vi "LPCA Interface Front Panel Update.vi"(6 "Resistance":refnum<vi>, 7 "index":i32, 8 "error in (no error)":errorcluster, 9 "Cluster":T1={"Queue Array"=[], "Queue Element"={"state"="", "data"=variant}, "System Event"=refnum, "System Event RefNum"=refnum, "Queue List"=[], "LPCA COM"="", "Rotating"=FALSE, "PrecorAI"="", "T_0 Index"=0, "Bar Graph X"=[], "Channels"=[], "Active Indicies"=[], "Active Channels"=[], "Sample Frequency"=0.0, "Resistance Sweep"=[], "RPM Sweep"=[], "Load Sweep"=[], "Step Height Sweep"=[], "Range Sweep"=[], "A Counter"=0, "B Counter"=0, "C Counter"=0, "#A"=0, "#B"=0, "#C"=0, "Current RPM"=0.0, "Current Resistance"=0, "Current Range"=0, "Current Step Height"=0, "Load Bank"=enum."OFF", "Cfg Cntrls"=[], "T_Monitor Indices"=[], "Thermal Limit"=0, "Thermal Resume"=0, "Timer Reset"=FALSE, "Stop Time"=0.0, "Autotest"=FALSE, "Pulsed RPM Capture"=FALSE, "Get Sample"=FALSE, "Last State"="", "Reset Timeout"=FALSE, "Ctrl Refs"={"Test Details"=refnum, "Save Config"=refnum, "Load Config"=refnum, "Path"=refnum, "Snapshot"=refnum, "SS#"=refnum, "Resistance"=refnum, "RPM Target"=refnum, "Spin"=refnum, "Load Bank"=refnum, "Start Test"=refnum, "Pause Test"=refnum, "Load Sweep"=refnum, "RPM Sweep"=refnum, "Resistance Sweep"=refnum, "Filters"=refnum, "Sample Frequency"=refnum, "Data Setup"=refnum, "Pause"=refnum, "Stop Time"=refnum, "S Period"=refnum, "Range"=refnum, "Step Height"=refnum, "Step Height Sweep"=refnum, "Range Sweep"=refnum, "Available Tests"=refnum, "RPM Graph"=refnum, "RPM Knob"=refnum, "FanMode"=refnum, "Fan Mode LED Array"=refnum, "Thermal Equilibrium"=refnum, "Data Display"=refnum, "LPCA Error"=refnum, "LPCA Ramp"=refnum, "LPCA Range"=refnum, "LPCA Resistance"=refnum}, "Pulse Waveform"={"t0"=timestamp(0 s since 1904-01-01), "dt"=1.0, "Y"=[]}, "Snapshot"={"Test Details"="test", "Version"="test", "Date"=timestamp(3493915594.3018084 s since 1904-01-01), "Selected Test"="man", "Snapshot Number"=0, "Time"=timestamp(3493915602.7292905 s since 1904-01-01), "Resistance Setpoint"="1", "RPM Setpoint"="20", "Range Setpoint"="", "Step Height Setpoint"="", "Load Bank Setpoint"="15", "Measurement Headers"="a,b,c,1,2,3", "Measurements"="1,2,3,4,5,6,7,8", "A"=0, "B"=0, "C"=0, "Raw Data"=[], "Available Tests"=enum."Manual", "Resistance List"="", "RPM List"="", "Load Bank List"="", "Range List"="", "Step Height List"="", "FanMode Setpoint"=enum."Auto"}, "Sample Period"=0.0, "OverTemp"=FALSE, "Available Tests"=enum."Manual", "FanMode"=enum."Auto", "Fan Mode LED Array"=[FALSE, TRUE, FALSE], "Thermal\nEquilibrium "=FALSE, "Equilibrium Stop"=FALSE, "AvgDegChg"=[]} {"Snapshot"."Time" format="%<%H:%M:%S>T"; "Snapshot"."Date" format="%<%m/%d/%Y>T"}, 10 "String":refnum<vi>) -> ()   [LabVIEW 2017]
uses:
  Controls/LPCA Commands.ctl
  <vilib>/regexp/Match Regular Expression.xnode
  <vilib>/Instr/_visa.llb/VISA Configure Serial Port (Instr).vi
  Code Library/Queue Element.ctl
  Code Library/Queue References Array.ctl
  Controls/Test TypeDef.ctl
  Controls/Available Tests.ctl
  Controls/Snapshot Typedef.ctl
  Controls/Load Bank.ctl
  Controls/FanMode.ctl
panel:
  out "return count":u32
  out "Stop?":bool=TRUE
  out "VISA resource name out":refnum<visa-resource-name>
  out "before match":string
  out "number of replacements":i32
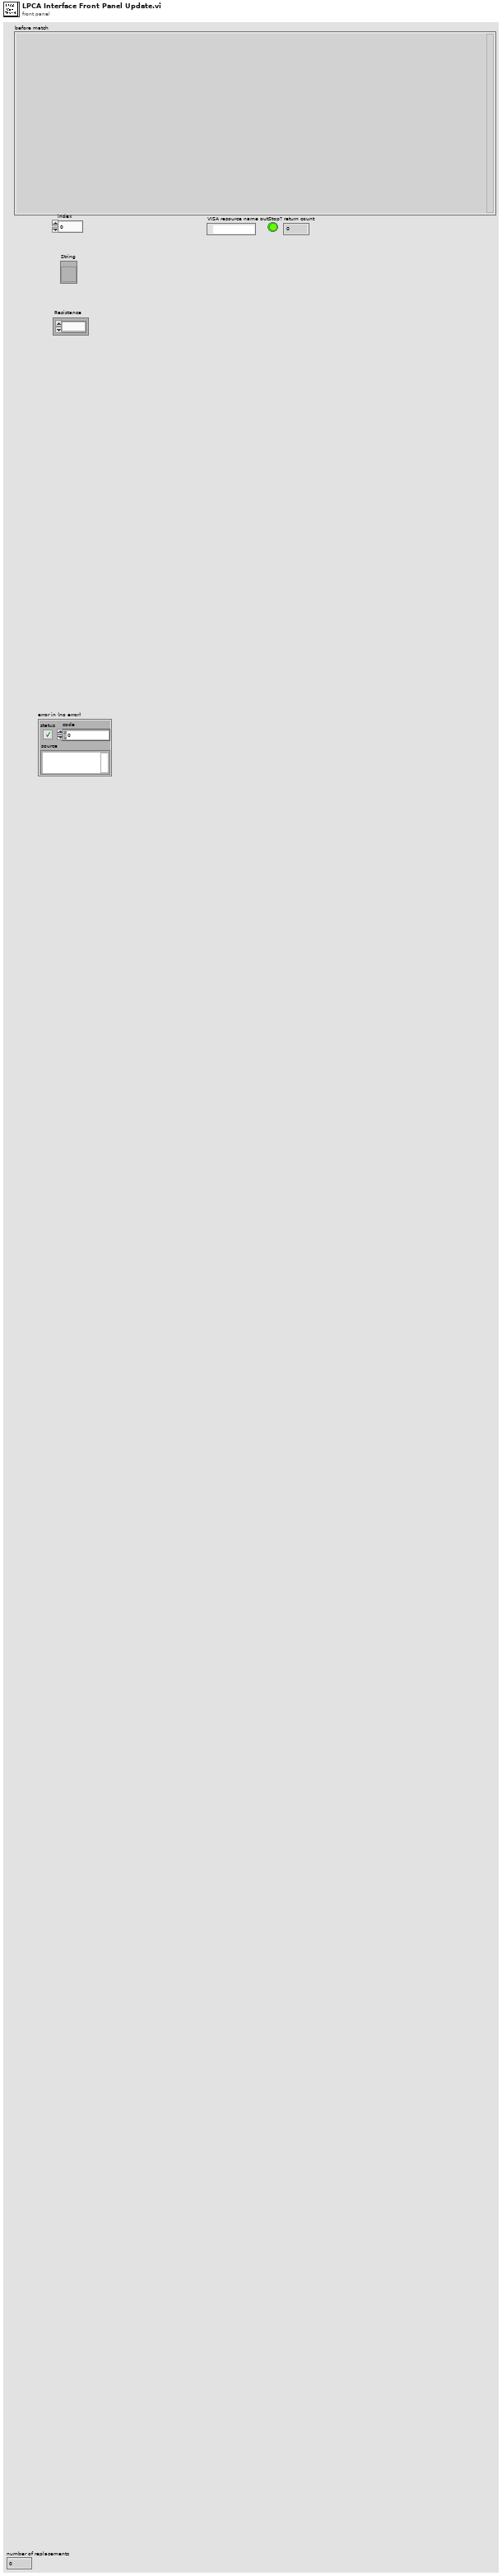
[diagram p1: front panel]
types:
  T1 = typedef "Test TypeDef.ctl" = cluster{"Queue Array":T2, "Queue Element":T3, "System Event":refnum<user-event>, "System Event RefNum":refnum<event-registration>, "Queue List":string[], "LPCA COM":refnum<visa-resource-name>, "Rotating":bool, "PrecorAI":refnum<k21>, "T_0 Index":i32, "Bar Graph X":i32[], "Channels":string[], "Active Indicies":i32[], "Active Channels":string[][], "Sample Frequency":dbl, "Resistance Sweep":string[], "RPM Sweep":string[], "Load Sweep":string[], "Step Height Sweep":string[], "Range Sweep":string[], "A Counter":i32, "B Counter":i32, "C Counter":i32, "#A":i32, "#B":i32, "#C":i32, "Current RPM":dbl, "Current Resistance":u32, "Current Range":u32, "Current Step Height":u32, "Load Bank":T4, "Cfg Cntrls":refnum<vi>[], "T_Monitor Indices":i32[], "Thermal Limit":i32, "Thermal Resume":i32, "Timer Reset":bool, "Stop Time":dbl, "Autotest":bool, "Pulsed RPM Capture":bool, "Get Sample":bool, "Last State":string, "Reset Timeout":bool, "Ctrl Refs":cluster{"Test Details":refnum<vi>, "Save Config":refnum<vi>, "Load Config":refnum<vi>, "Path":refnum<vi>, "Snapshot":refnum<vi>, "SS#":refnum<vi>, "Resistance":refnum<vi>, "RPM Target":refnum<vi>, "Spin":refnum<vi>, "Load Bank":refnum<vi>, "Start Test":refnum<vi>, "Pause Test":refnum<vi>, "Load Sweep":refnum<vi>, "RPM Sweep":refnum<vi>, "Resistance Sweep":refnum<vi>, "Filters":refnum<vi>, "Sample Frequency":refnum<vi>, "Data Setup":refnum<vi>, "Pause":refnum<vi>, "Stop Time":refnum<vi>, "S Period":refnum<vi>, "Range":refnum<vi>, "Step Height":refnum<vi>, "Step Height Sweep":refnum<vi>, "Range Sweep":refnum<vi>, "Available Tests":refnum<vi>, "RPM Graph":refnum<vi>, "RPM Knob":refnum<vi>, "FanMode":refnum<vi>, "Fan Mode LED Array":refnum<vi>, "Thermal Equilibrium":refnum<vi>, "Data Display":refnum<vi>, "LPCA Error":refnum<vi>, "LPCA Ramp":refnum<vi>, "LPCA Range":refnum<vi>, "LPCA Resistance":refnum<vi>}, "Pulse Waveform":waveform(dbl), "Snapshot":T5, "Sample Period":dbl, "OverTemp":bool, "Available Tests":T6, "FanMode":T7, "Fan Mode LED Array":bool[], "Thermal\nEquilibrium ":bool, "Equilibrium Stop":bool, "AvgDegChg":dbl[]}
  T2 = typedef "Queue References Array.ctl" = refnum<queue>[]
  T3 = typedef "Queue Element.ctl" = cluster{"state":string, "data":variant}
  T4 = typedef "Load Bank.ctl" = enum16{"OFF", "50", "25", "16.7", "12.5", "10.0", "8.3", "7.1", "6.3", "5.6", "5.0", "4.5", "4.2", "3.8", "3.6", "3.3", "3.1"}
  T5 = typedef "Snapshot Typedef.ctl" = cluster{"Test Details":string, "Version":string, "Date":timestamp, "Selected Test":string, "Snapshot Number":u16, "Time":timestamp, "Resistance Setpoint":string, "RPM Setpoint":string, "Range Setpoint":string, "Step Height Setpoint":string, "Load Bank Setpoint":string, "Measurement Headers":string, "Measurements":string, "A":i32, "B":i32, "C":i32, "Raw Data":string[][], "Available Tests":T6, "Resistance List":string, "RPM List":string, "Load Bank List":string, "Range List":string, "Step Height List":string, "FanMode Setpoint":T7}
  T6 = typedef "Available Tests.ctl" = enum16{"Manual", "EFX Brake Torque", "Generator Torque", "EFX Brake Thermal", "Generator Thermal", "Pulsed RPM", "AMT Brake Torque", "Bike Brake Torque", "AMT Brake Thermal", "Bike Brake Thermal"}
  T7 = typedef "FanMode.ctl" = enum16{"On", "Off", "Auto"}
  T8 = typedef "LPCA Commands.ctl" = enum16{"RSET", "stop", "rpmh", "rpml", "prpm", "rpm", "res", "rng", "tmp1", "tmp2", "err", "ramp"}
  T9 = cluster{"Test Details":refnum<vi>, "Save Config":refnum<vi>, "Load Config":refnum<vi>, "Path":refnum<vi>, "Snapshot":refnum<vi>, "SS#":refnum<vi>, "Resistance":refnum<vi>, "RPM Target":refnum<vi>, "Spin":refnum<vi>, "Load Bank":refnum<vi>, "Start Test":refnum<vi>, "Pause Test":refnum<vi>, "Load Sweep":refnum<vi>, "RPM Sweep":refnum<vi>, "Resistance Sweep":refnum<vi>, "Filters":refnum<vi>, "Sample Frequency":refnum<vi>, "Data Setup":refnum<vi>, "Pause":refnum<vi>, "Stop Time":refnum<vi>, "S Period":refnum<vi>, "Range":refnum<vi>, "Step Height":refnum<vi>, "Step Height Sweep":refnum<vi>, "Range Sweep":refnum<vi>, "Available Tests":refnum<vi>, "RPM Graph":refnum<vi>, "RPM Knob":refnum<vi>, "FanMode":refnum<vi>, "Fan Mode LED Array":refnum<vi>, "Thermal Equilibrium":refnum<vi>, "Data Display":refnum<vi>, "LPCA Error":refnum<vi>, "LPCA Ramp":refnum<vi>, "LPCA Range":refnum<vi>, "LPCA Resistance":refnum<vi>}
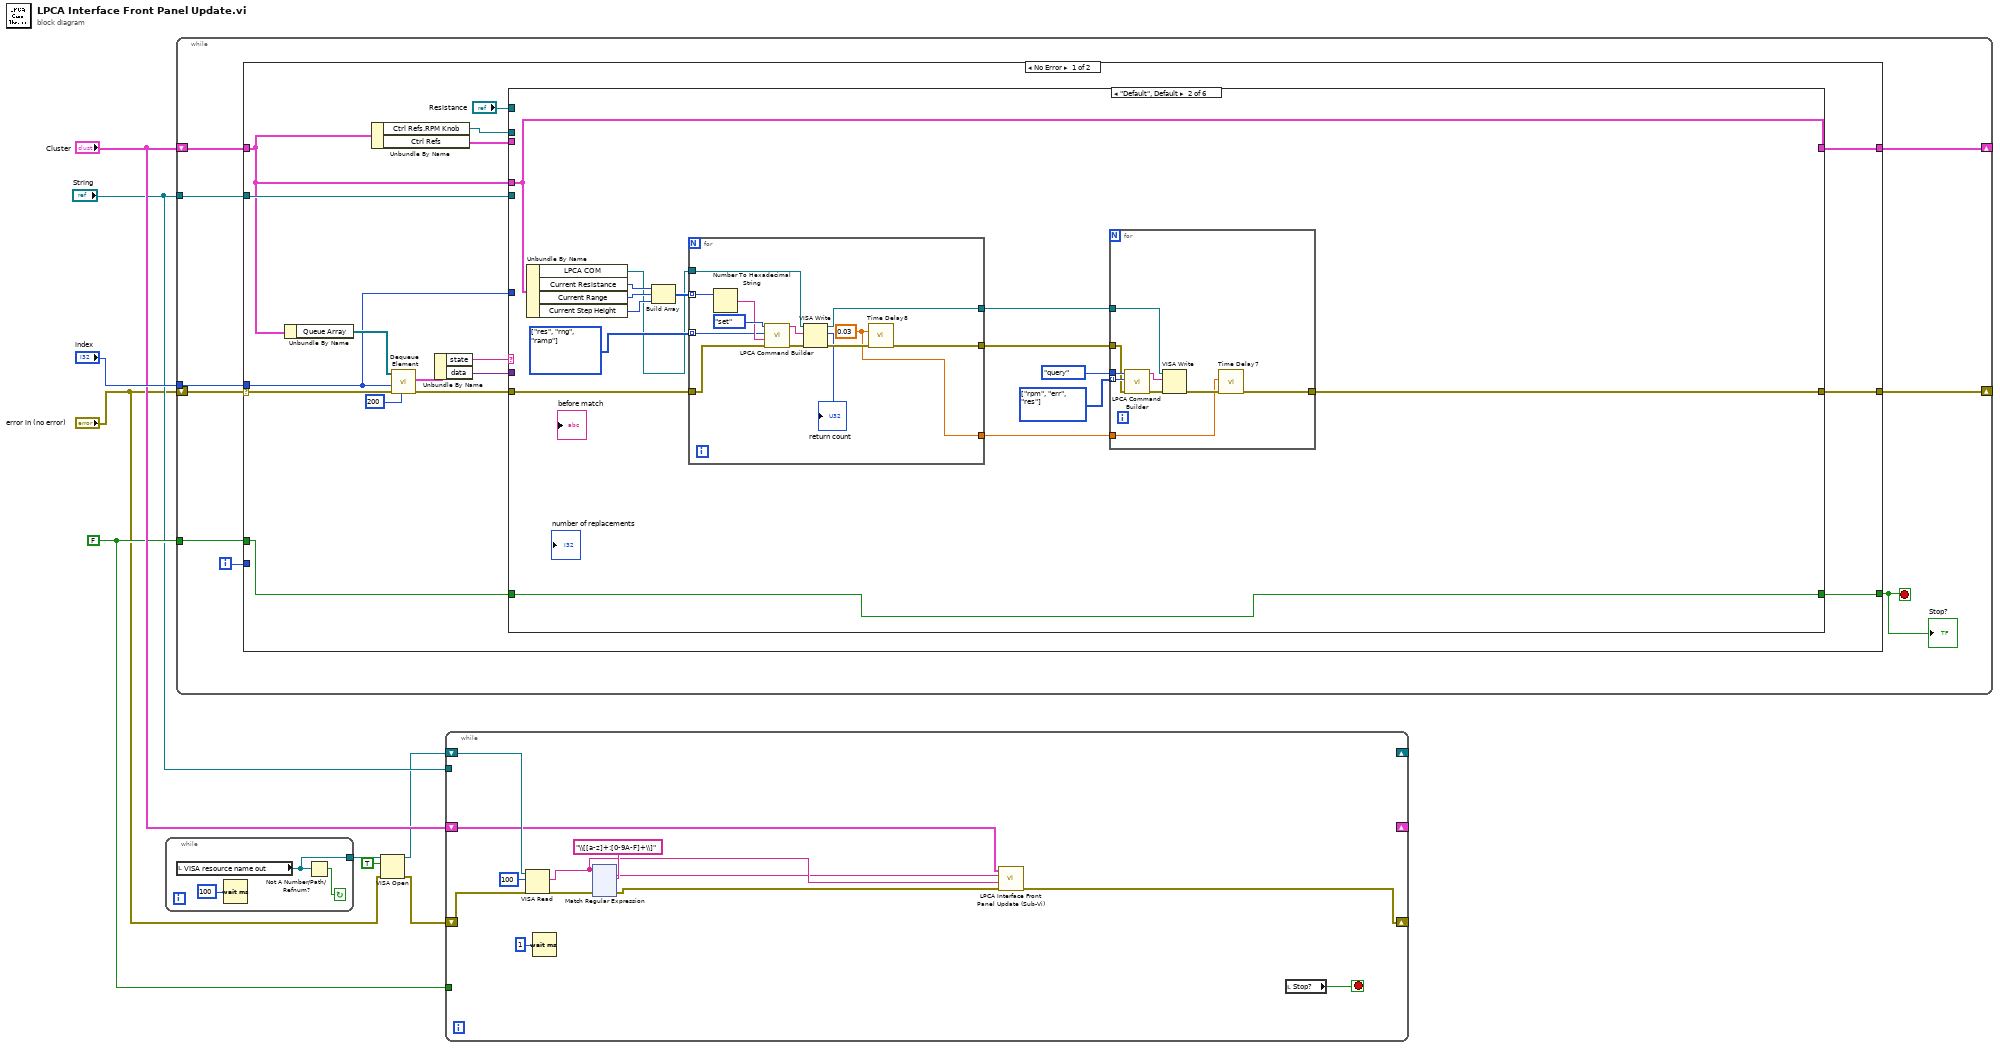
[diagram p0: block diagram]
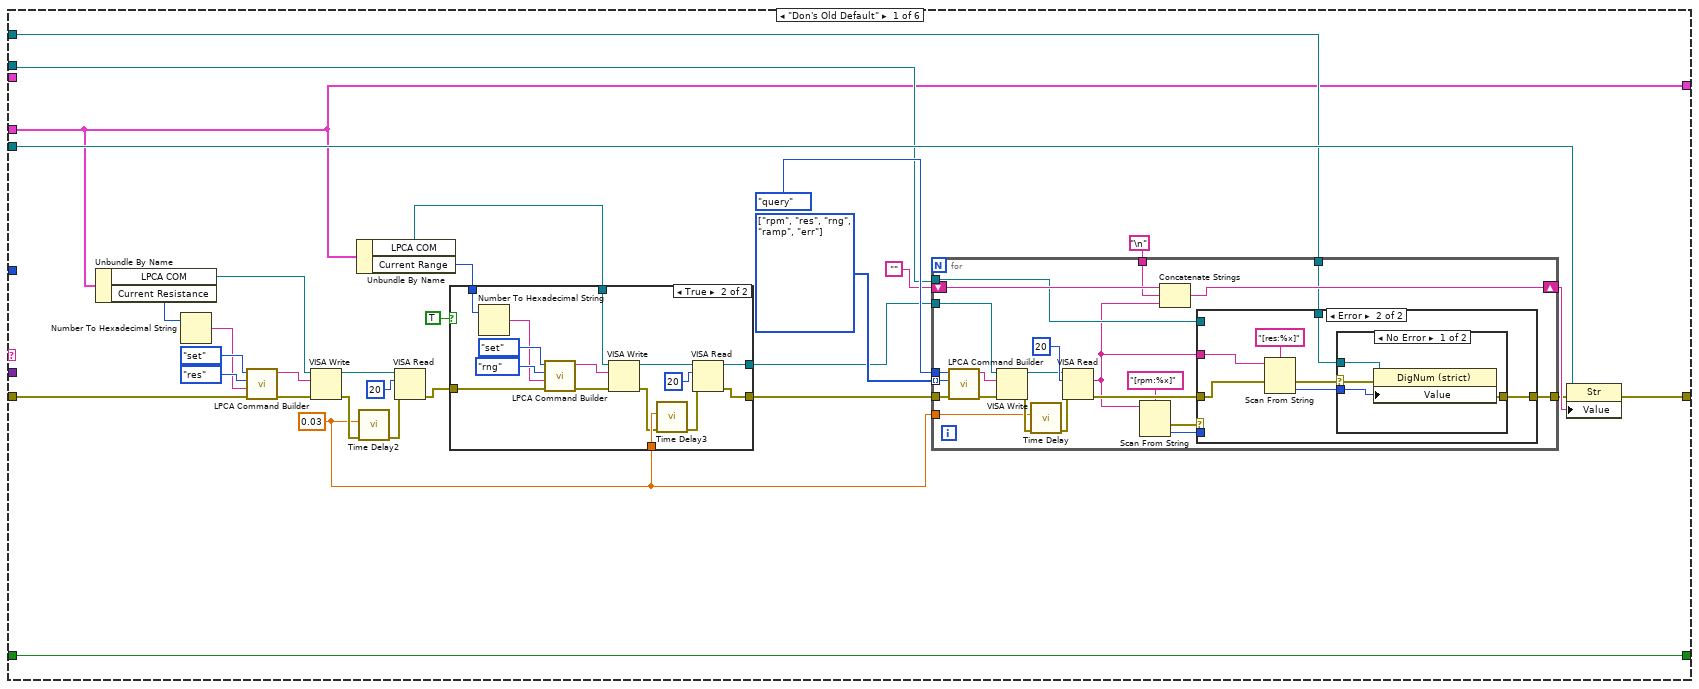
[diagram p2: hidden frame]
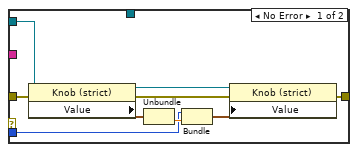
[diagram p4: hidden frame]
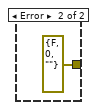
[diagram p5: hidden frame]
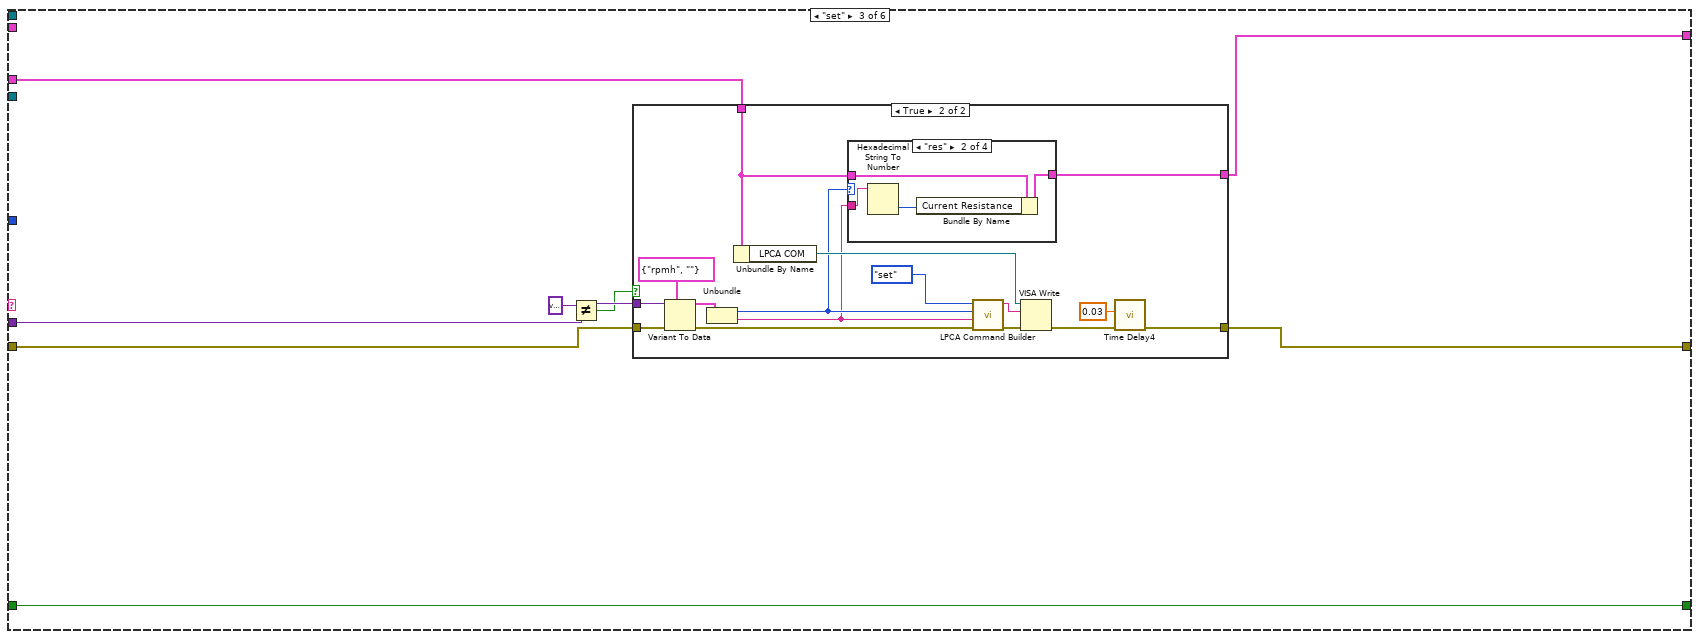
[diagram p6: hidden frame]
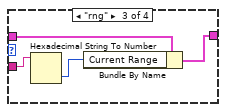
[diagram p9: hidden frame]
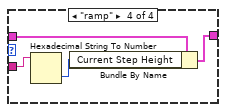
[diagram p10: hidden frame]
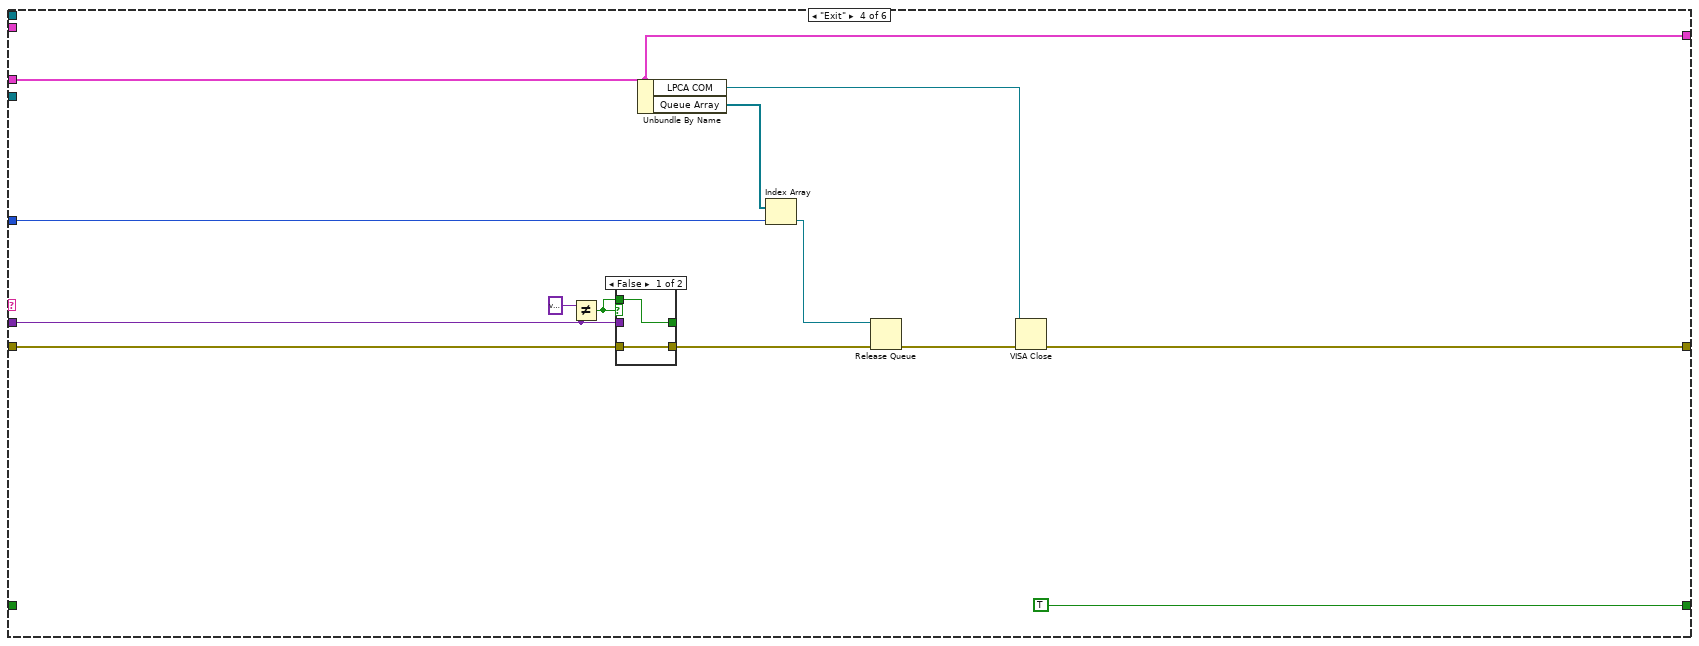
[diagram p11: hidden frame]
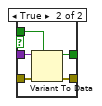
[diagram p12: hidden frame]
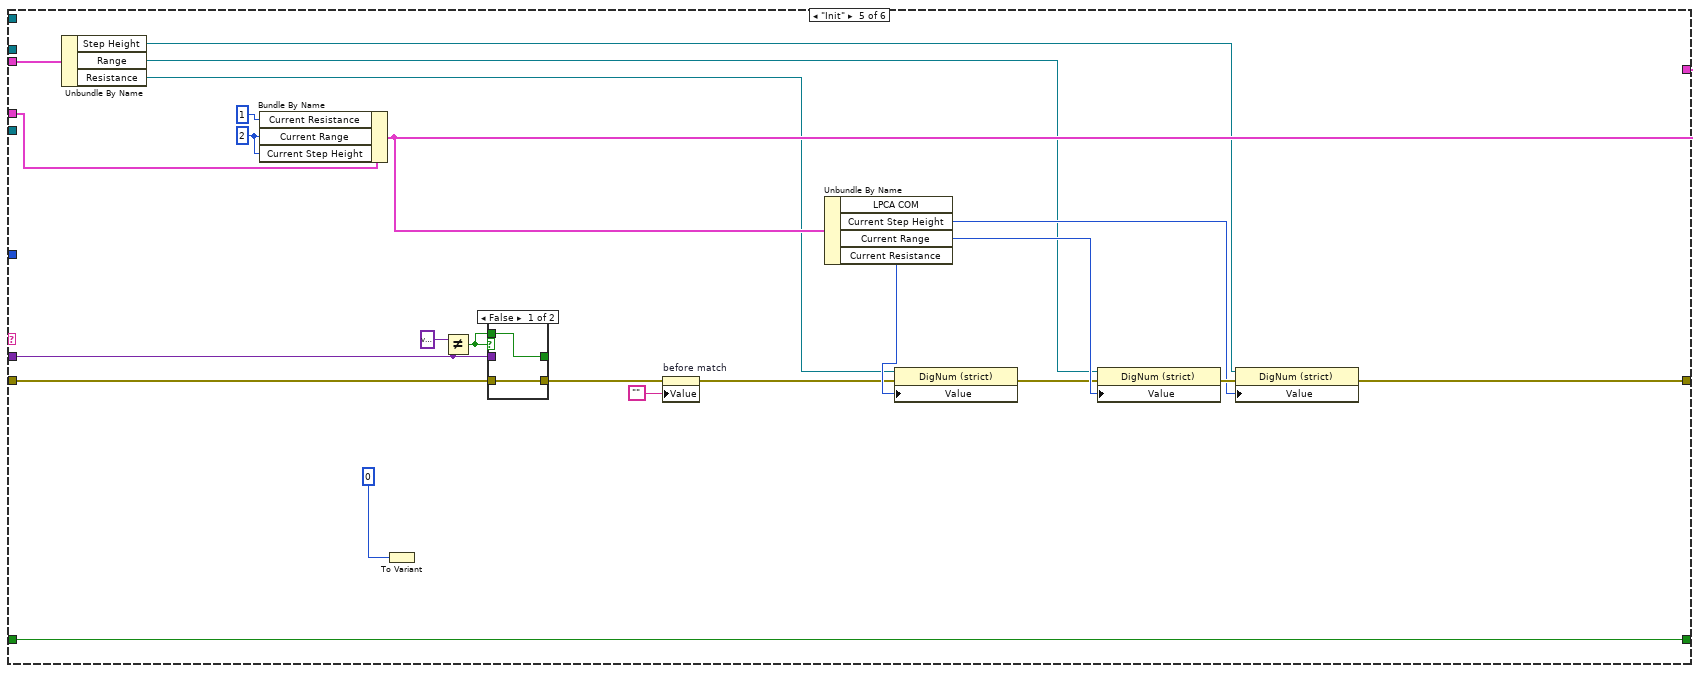
[diagram p13: hidden frame]
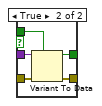
[diagram p14: hidden frame]
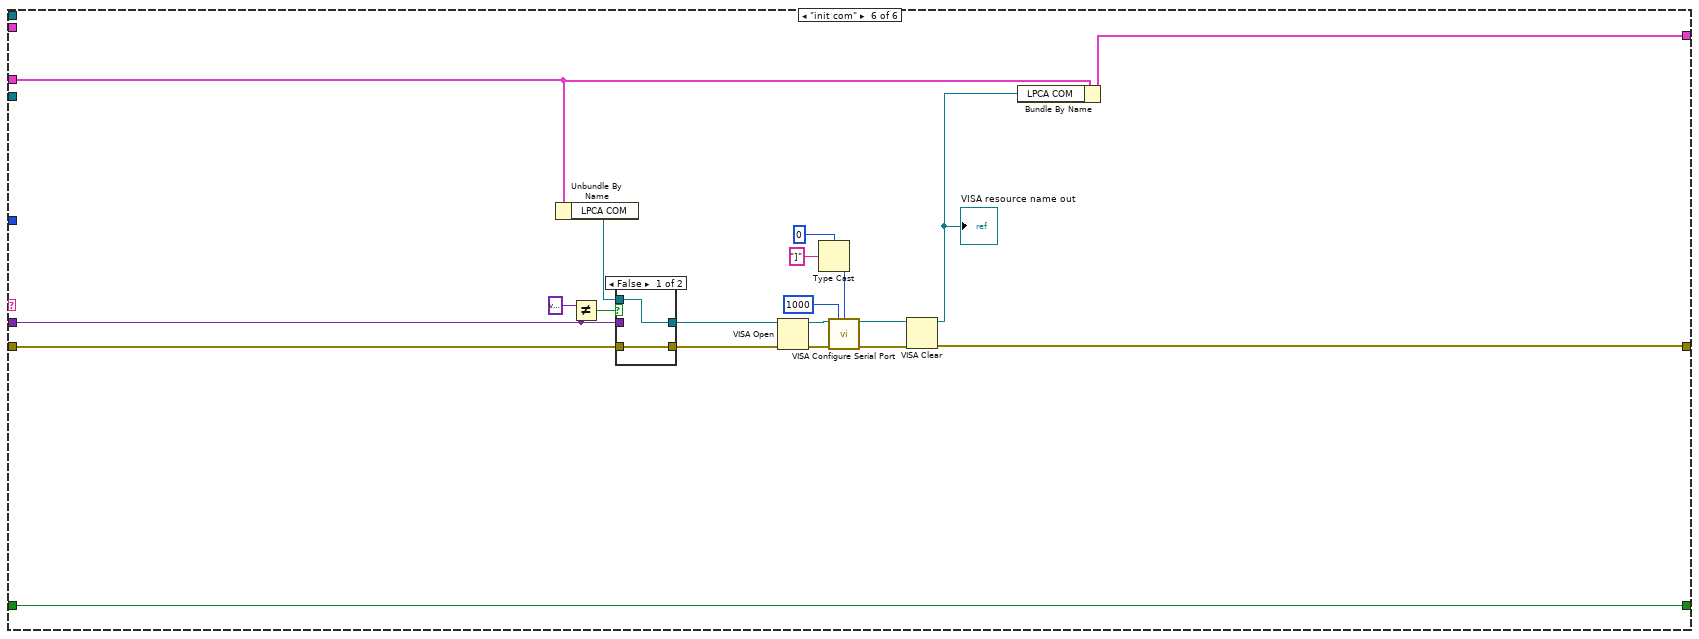
[diagram p15: hidden frame]
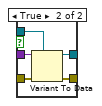
[diagram p16: hidden frame]
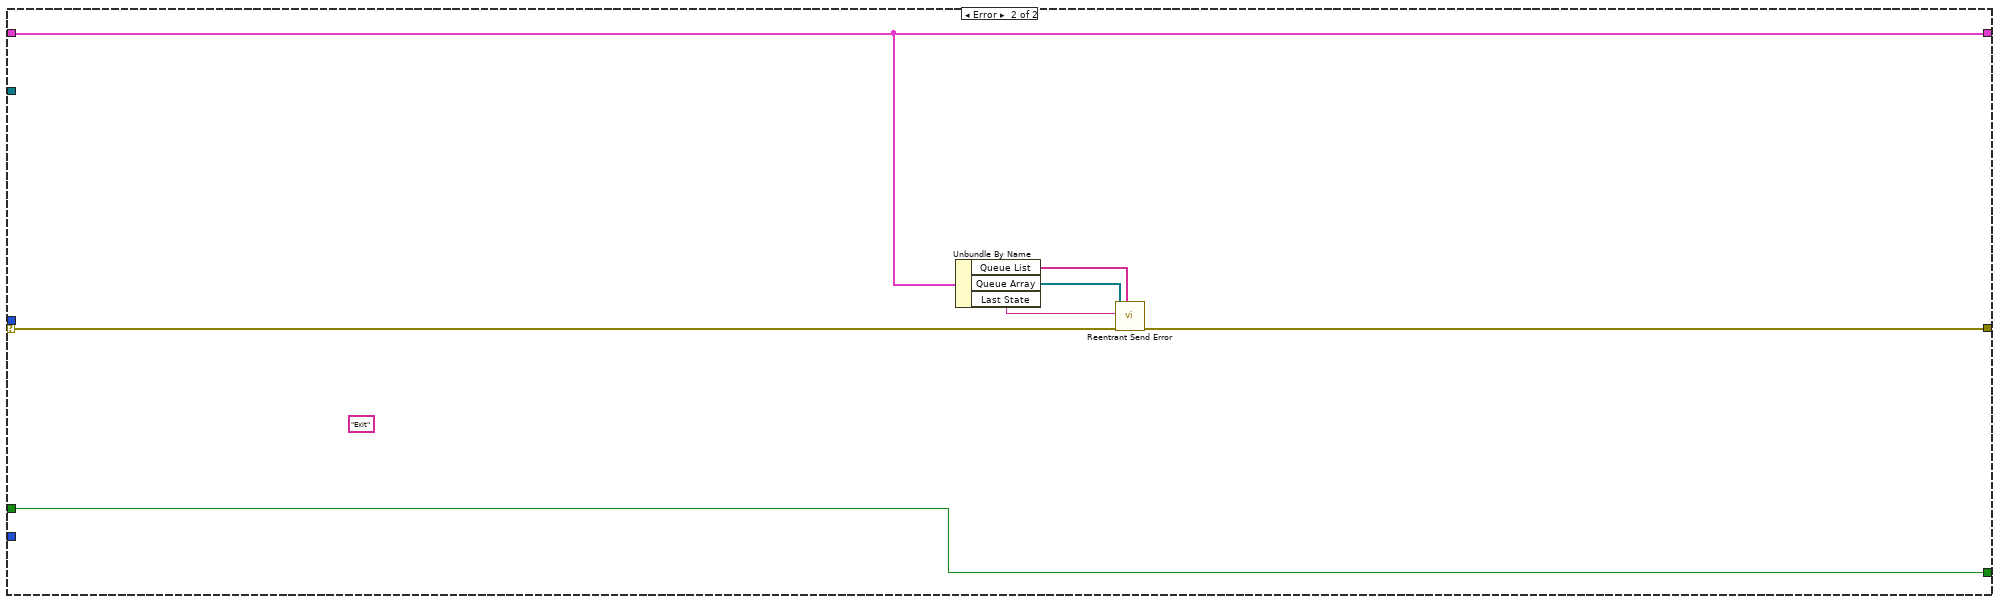
[diagram p17: hidden frame]
diagram:
  w7 = FALSE ("Boolean")
  n1 = while {
    tunnel: [w10] -> w5
    stop <- w11 continue-if-true
    n2 = local read "VISA resource name out"() -> (w10:refnum<visa-resource-name>)
    n3 = Wait (ms)(milliseconds to wait=u32 100) -> ()  [unwired: 1 out]
    n4 = Not A Number/Path/Refnum?(number/path/refnum=w10) -> (NaN/Path/Refnum?=w11:bool)
  }
  n5 = while {
    shift-right: [w17] -> _
    shift-left: "Cluster" -> [w21]
    tunnel: w7 -> [w18]
    shift-right: [w19] -> _
    shift-left: "error in (no error)" -> [w20]
    tunnel: "index" -> [w16]
    tunnel: "String" -> [w15]
    i -> [w14]
    stop <- w13 stop-if-true
    n6 = case shown="No Error" w20 {
      selector: w20 -> [w36 w285]
      tunnel: w21 -> [w23 w283]
      tunnel: [w34 w284] -> w19
      tunnel: w18 -> [w33 w289]
      tunnel: [w32 w289] -> w13
      tunnel: [w30 w283] -> w17
      tunnel: w16 -> [w26 _]
      tunnel: w15 -> [w29 _]
      tunnel: w14 -> [_ _]
      frame No Error {
        n7 = Unbundle By Name(w23) -> ("Queue Array"=w38:T2)
        n8 = Unbundle By Name(w23) -> ("Ctrl Refs.RPM Knob"=w25:refnum<vi>, "Ctrl Refs"=w24:T9)
        n9 = call "Dequeue Element.vi"("timeout in ms (-1)"=200, "error in (no error)"=w36, "index"=w26, "Queue Array"=w38) -> ("error out"=w35:errorcluster, "Queue Element"=w28:T3)  [unwired: 5 in, 1 out]
        n10 = Unbundle By Name(w28) -> ("state"=w22:string, "data"=w31:variant)
        n11 = case shown="\"Default\", Default" w22 {
          tunnel: w35 -> [w49 w133 w173 w218 w247 w274]
          tunnel: [w68 w130 w170 w211 w226 w256] -> w34
          tunnel: w33 -> [w69 w144 w174 _ w248 w275]
          tunnel: [w69 w144 w174 TRUE ("Boolean") w248 w275] -> w32
          tunnel: w31 -> [_ _ w171 w216 w245 w272]
          tunnel: [w43 w132 w167 w214 w236 w270] -> w30
          tunnel: w23 -> [w43 w132 w168 w214 w239 w262]
          tunnel: w29 -> [w66 _ _ _ _ _]
          tunnel: w25 -> [w48 _ _ _ _ _]
          tunnel: "Resistance" -> [w47 _ _ _ _ _]
          tunnel: w26 -> [_ _ _ w208 _ _]
          tunnel: w24 -> [_ _ _ _ w235 _]
          frame "Don's Old Default" {
            w53 = T8[] [enum."rpm", enum."res", enum."rng", enum."ramp", enum."err"] items=["RSET", "stop", "rpmh", "rpml", "prpm", "rpm", "res", "rng", "tmp1", "tmp2", "err", "ramp"]
            w46 = 0.03 ("Delay Time (s)")
            n12 = Unbundle By Name(w43) -> ("LPCA COM"=w67:refnum<visa-resource-name>, "Current Resistance"=w65:u32)
            n13 = Number To Hexadecimal String(2:w65) -> (0:w55:string)  [unwired: 1 in]
            n14 = call "LPCA Command Builder.vi"("error in (no error)"=w49, "Data"=w55, "LPCA Command"=LPCA_Commands."res", "Mode"=enum16{"set", "query"}."set") -> ("error out"=w56:errorcluster, "String"=w57:string)  [unwired: 6 in]
            n15 = VISA Write(VISA resource name=w67, write buffer=w57, error in (no error)=w56) -> (VISA resource name out=w51:refnum<visa-resource-name>, error out=w54:errorcluster)  [unwired: 1 out]
            n16 = Unbundle By Name(w43) -> ("LPCA COM"=w41:refnum<visa-resource-name>, "Current Range"=w44:u32)
            n17 = call "Time Delay2"("error in (no error)"=w54, "Delay Time (s)"=w46) -> ("error out"=w50:errorcluster)  [unwired: 9 in]
            n18 = VISA Read(VISA resource name=w51, byte count=u32 20, error in (no error)=w50) -> (error out=w45:errorcluster)  [unwired: 3 out]
            n19 = case shown="True" TRUE {
              tunnel: w46 -> [_ w80]
              tunnel: w45 -> [w71 w79]
              tunnel: w44 -> [_ w78]
              tunnel: [w71 w75] -> w42
              tunnel: w41 -> [w70 w73]
              tunnel: [w70 w72] -> w40
              frame False {
              }
              frame True {
                n20 = Number To Hexadecimal String(2:w78) -> (0:w74:string)  [unwired: 1 in]
                n21 = call "LPCA Command Builder.vi"("error in (no error)"=w79, "Data"=w74, "LPCA Command"=LPCA_Commands."rng", "Mode"=enum16{"set", "query"}."set") -> ("error out"=w83:errorcluster, "String"=w84:string)  [unwired: 6 in]
                n22 = VISA Write(VISA resource name=w73, write buffer=w84, error in (no error)=w83) -> (VISA resource name out=w81:refnum<visa-resource-name>, error out=w77:errorcluster)  [unwired: 1 out]
                n23 = call "Time Delay3"("error in (no error)"=w77, "Delay Time (s)"=w80) -> ("error out"=w76:errorcluster)  [unwired: 9 in]
                n24 = VISA Read(VISA resource name=w81, byte count=u32 20, error in (no error)=w76) -> (VISA resource name out=w72:refnum<visa-resource-name>, error out=w75:errorcluster)  [unwired: 2 out]
              }
            }
            n25 = for {
              tunnel: enum16{"set", "query"}."query" ("Mode") -> [w104]
              tunnel: w42 -> [w103]
              tunnel: [w96] -> w60
              tunnel: w40 -> [w102]
              tunnel: w53 -> [w98] mode=indexing
              shift-right: [w101] -> w61
              shift-left: "" -> [w100]
              tunnel: "\n" -> [w99]
              tunnel: w48 -> [w95]
              tunnel: w47 -> [w88]
              tunnel: w46 -> [w87]
              n26 = call "LPCA Command Builder.vi"("error in (no error)"=w103, "LPCA Command"=w98, "Mode"=w104) -> ("error out"=w107:errorcluster, "String"=w108:string)  [unwired: 7 in]
              n27 = VISA Write(VISA resource name=w102, write buffer=w108, error in (no error)=w107) -> (VISA resource name out=w105:refnum<visa-resource-name>, error out=w90:errorcluster)  [unwired: 1 out]
              n28 = call "Time Delay"("error in (no error)"=w90, "Delay Time (s)"=w87) -> ("error out"=w89:errorcluster)  [unwired: 9 in]
              n29 = VISA Read(VISA resource name=w105, byte count=u32 20, error in (no error)=w89) -> (read buffer=w93:string, error out=w97:errorcluster)  [unwired: 2 out]
              n30 = Scan From String(format string="[rpm:%x]", input string=w93) -> (error out=w92:errorcluster, output 1=w91:u32)  [unwired: 3 in, 2 out]
              n31 = Concatenate Strings(w100, w99, w93) -> (w101:string)
              n32 = case shown="Error" w92 {
                tunnel: w97 -> [w116 w118]
                tunnel: [w117 w119] -> w96
                tunnel: w95 -> [w115 _]
                tunnel: w93 -> [_ w123]
                tunnel: w91 -> [w109 _]
                tunnel: w88 -> [_ w120]
                frame No Error {
                  n33 = property class="Knob (strict)"(reference=w115, error in=w116) -> (reference out=w113:refnum<vi>, error out=w114:errorcluster, "Value"=w110:cluster{dbl, dbl})
                  n34 = Unbundle(w110) -> (w111:dbl)  [unwired: 1 out]
                  n35 = Bundle(w109, w111) -> (w112:cluster{u32, dbl})  [unwired: 1 in]
                  n36 = property class="Knob (strict)"(reference=w113, error in=w114, "Value"=w112) -> (error out=w117:errorcluster)  [unwired: 1 out]
                }
                frame Error {
                  n37 = Scan From String(format string="[res:%x]", input string=w123, error in=w118) -> (error out=w122:errorcluster, output 1=w121:u32)  [unwired: 2 in, 2 out]
                  n38 = case shown="No Error" w122 {
                    selector: w122 -> [w128 _]
                    tunnel: w121 -> [w125 _]
                    tunnel: w120 -> [w126 _]
                    tunnel: [w127 errorcluster {"status"=FALSE, "code"=0, "source"=""} ("error out")] -> w119
                    frame No Error {
                      n39 = property class="DigNum (strict)"(reference=w126, error in=w128, "Value"=w125) -> (error out=w127:errorcluster)  [unwired: 1 out]
                    }
                    frame Error {
                    }
                  }
                }
              }
            }
            n40 = property class="Str"(reference=w66, error in=w60, "Value"=w61) -> (error out=w68:errorcluster)  [unwired: 1 out]
          }
          frame "Default", Default {
            w135 = T8[] [enum."rpm", enum."err", enum."res"] items=["RSET", "stop", "rpmh", "rpml", "prpm", "rpm", "res", "rng", "tmp1", "tmp2", "err", "ramp"]
            w138 = T8[] [enum."res", enum."rng", enum."ramp"] items=["RSET", "stop", "rpmh", "rpml", "prpm", "rpm", "res", "rng", "tmp1", "tmp2", "err", "ramp"]
            n41 = Unbundle By Name(w132) -> ("LPCA COM"=w134:refnum<visa-resource-name>, "Current Resistance"=w142:u32, "Current Range"=w141:u32, "Current Step Height"=w140:u32)
            n42 = Build Array(w142, w141, w140) -> (w139:u32[])
            n43 = for {
              tunnel: w139 -> [w152] mode=indexing
              tunnel: w134 -> [w153]
              tunnel: w138 -> [w151] mode=indexing
              tunnel: [w147] -> w137
              tunnel: w133 -> [w149]
              tunnel: [w150] -> w136
              tunnel: [w146] -> w131
              w150 = 0.03 ("Delay Time (s)")
              n44 = Number To Hexadecimal String(2:w152) -> (0:w155:string)  [unwired: 1 in]
              n45 = call "LPCA Command Builder.vi"("error in (no error)"=w149, "Data"=w155, "LPCA Command"=w151, "Mode"=enum16{"set", "query"}."set") -> ("error out"=w156:errorcluster, "String"=w148:string)  [unwired: 6 in]
              n46 = VISA Write(VISA resource name=w153, write buffer=w148, error in (no error)=w156) -> (VISA resource name out=w147:refnum<visa-resource-name>, return count=→"return count":u32, error out=w154:errorcluster)
              n47 = call "Time Delay8"("error in (no error)"=w154, "Delay Time (s)"=w150) -> ("error out"=w146:errorcluster)  [unwired: 9 in]
            }
            n48 = for {
              tunnel: enum16{"set", "query"}."query" ("Mode") -> [w165]
              tunnel: w137 -> [w164]
              tunnel: w135 -> [w163] mode=indexing
              tunnel: w136 -> [w161]
              tunnel: [w158] -> w130
              tunnel: w131 -> [w159]
              n49 = call "LPCA Command Builder.vi"("error in (no error)"=w159, "LPCA Command"=w163, "Mode"=w165) -> ("error out"=w166:errorcluster, "String"=w160:string)  [unwired: 7 in]
              n50 = VISA Write(VISA resource name=w164, write buffer=w160, error in (no error)=w166) -> (error out=w162:errorcluster)  [unwired: 2 out]
              n51 = call "Time Delay7"("error in (no error)"=w162, "Delay Time (s)"=w161) -> ("error out"=w158:errorcluster)  [unwired: 9 in]
            }
          }
          frame "set" {
            n52 = Not Equal?(x=variant, y=w171) -> (x != y?=w169:bool)
            n53 = case shown="True" w169 {
              tunnel: w173 -> [w176 w192]
              tunnel: w171 -> [_ w191]
              tunnel: w168 -> [w175 w182]
              tunnel: [w176 w177] -> w170
              tunnel: [w175 w180] -> w167
              frame False {
              }
              frame True {
                n54 = Variant To Data(error in=w192, type=cluster{T8, string} {enum."rpmh", ""}, Variant=w191) -> (data=w184:cluster{T8, string}, error out=w189:errorcluster)
                n55 = Unbundle(w184) -> (w183:T8, w181:string)
                n56 = Unbundle By Name(w182) -> ("LPCA COM"=w190:refnum<visa-resource-name>)
                n57 = case shown="\"res\"" w183 {
                  tunnel: w182 -> [w193 w197 w201 w205]
                  tunnel: w181 -> [_ w195 w199 w203]
                  tunnel: [w193 w196 w200 w204] -> w180
                  frame "RSET", Default {
                  }
                  frame "res" {
                    n58 = Hexadecimal String To Number(string=w195) -> (number=w194:u32)  [unwired: 2 in, 1 out]
                    n59 = Bundle By Name(cluster=w197, "Current Resistance"=w194) -> (w196:T1)
                  }
                  frame "rng" {
                    n60 = Hexadecimal String To Number(string=w199) -> (number=w198:u32)  [unwired: 2 in, 1 out]
                    n61 = Bundle By Name(cluster=w201, "Current Range"=w198) -> (w200:T1)
                  }
                  frame "ramp" {
                    n62 = Hexadecimal String To Number(string=w203) -> (number=w202:u32)  [unwired: 2 in, 1 out]
                    n63 = Bundle By Name(cluster=w205, "Current Step Height"=w202) -> (w204:T1)
                  }
                }
                n64 = call "LPCA Command Builder.vi"("error in (no error)"=w189, "Data"=w181, "LPCA Command"=w183, "Mode"=enum16{"set", "query"}."set") -> ("error out"=w186:errorcluster, "String"=w187:string)  [unwired: 6 in]
                n65 = VISA Write(VISA resource name=w190, write buffer=w187, error in (no error)=w186) -> (error out=w179:errorcluster)  [unwired: 2 out]
                n66 = call "Time Delay4"("error in (no error)"=w179, "Delay Time (s)"=0.03) -> ("error out"=w177:errorcluster)  [unwired: 9 in]
              }
            }
          }
          frame "Exit" {
            n67 = Not Equal?(x=variant, y=w216) -> (x != y?=w215:bool)
            n68 = case shown="False" w215 {
              tunnel: w218 -> [w220 w225]
              tunnel: [w220 w224] -> w213
              tunnel: w216 -> [_ w223]
              tunnel: [w219 w222] -> _
              tunnel: w215 -> [w219 w221]
              frame False {
              }
              frame True {
                n69 = Variant To Data(error in=w225, type=w221, Variant=w223) -> (data=w222:bool, error out=w224:errorcluster)
              }
            }
            n70 = Unbundle By Name(w214) -> ("LPCA COM"=w210:refnum<visa-resource-name>, "Queue Array"=w209:T2)
            n71 = Index Array(array=w209, index=w208) -> (element=w207:refnum<queue>)
            n72 = Release Queue(queue=w207, error in (no error)=w213) -> (error out=w212:errorcluster)  [unwired: 1 in, 2 out]
            n73 = VISA Close(VISA resource name=w210, error in (no error)=w212) -> (error out=w211:errorcluster)
          }
          frame "Init" {
            w242 = u32 2 ("Resistance Range")
            n74 = Unbundle By Name(w235) -> ("Step Height"=w233:refnum<vi>, "Range"=w234:refnum<vi>, "Resistance"=w230:refnum<vi>)
            n75 = Bundle By Name(cluster=w239, "Current Resistance"=u32 1, "Current Range"=w242, "Current Step Height"=w242) -> (w236:T1)
            n76 = To Variant(anything=u32 0 ("Resistance Range")) -> ()  [unwired: 1 out]
            n77 = Not Equal?(x=variant, y=w245) -> (x != y?=w244:bool)
            n78 = case shown="False" w244 {
              tunnel: w247 -> [w250 w255]
              tunnel: [w250 w254] -> w229
              tunnel: w245 -> [_ w253]
              tunnel: [w249 w252] -> _
              tunnel: w244 -> [w249 w251]
              frame False {
              }
              frame True {
                n79 = Variant To Data(error in=w255, type=w251, Variant=w253) -> (data=w252:bool, error out=w254:errorcluster)
              }
            }
            n80 = property on="before match" class="Str"(error in=w229, "Value"="") -> (error out=w228:errorcluster)  [unwired: 1 in, 1 out]
            n81 = Unbundle By Name(w236) -> ("Current Step Height"=w238:u32, "Current Range"=w237:u32, "Current Resistance"=w231:u32)  [unwired: 1 out]
            n82 = property class="DigNum (strict)"(reference=w230, error in=w228, "Value"=w231) -> (error out=w232:errorcluster)  [unwired: 1 out]
            n83 = property class="DigNum (strict)"(reference=w234, error in=w232, "Value"=w237) -> (error out=w240:errorcluster)  [unwired: 1 out]
            n84 = property class="DigNum (strict)"(reference=w233, error in=w240, "Value"=w238) -> (error out=w226:errorcluster)  [unwired: 1 out]
          }
          frame "init com" {
            n85 = Unbundle By Name(w262) -> ("LPCA COM"=w261:refnum<visa-resource-name>)
            n86 = Not Equal?(x=variant, y=w272) -> (x != y?=w271:bool)
            n87 = case shown="False" w271 {
              tunnel: w274 -> [w277 w282]
              tunnel: [w277 w281] -> w259
              tunnel: w272 -> [_ w280]
              tunnel: [w276 w279] -> w260
              tunnel: w261 -> [w276 w278]
              frame False {
              }
              frame True {
                n88 = Variant To Data(error in=w282, type=w278, Variant=w280) -> (data=w279:refnum<visa-resource-name>, error out=w281:errorcluster)
              }
            }
            n89 = VISA Open(error in (no error)=w259, VISA resource name=w260) -> (VISA resource name=w268:refnum<visa-resource-name>, error out=w269:errorcluster)  [unwired: 3 in]
            n90 = Type Cast(type=u8 0 ("termination char\n(0xA = '\\n' = LF)"), x="]") -> (*(type *) &x=w266:u8)
            n91 = call-poly "VISA Configure Serial Port"("VISA resource name"=w268, "timeout (10sec)"=u32 1000, "termination char\n(0xA = '\\n' = LF)"=w266, "error in (no error)"=w269) -> ("VISA resource name out"=w263:refnum<visa-resource-name>, "error out"=w257:errorcluster)  [unwired: 10 in]
            n92 = VISA Clear(VISA resource name=w263, error in (no error)=w257) -> (VISA resource name out=w258:refnum<visa-resource-name>, error out=w256:errorcluster)
            "VISA resource name out" <- w258
            n93 = Bundle By Name(cluster=w262, "LPCA COM"=w258) -> (w270:T1)
          }
        }
      }
      frame Error {
        (unwired) "Exit" ("state")
        n94 = Unbundle By Name(w283) -> ("Queue List"=w286:string[], "Queue Array"=w287:T2, "Last State"=w288:string)
        n95 = call "Reentrant Send Error.vi"("Queue Names"=w286, "error in (no error)"=w285, "Last State"=w288, "Queues"=w287) -> ("error out"=w284:errorcluster)  [unwired: 7 in]
      }
    }
    "Stop?" <- w13
  }
  n96 = VISA Open(duplicate session (F)=TRUE, error in (no error)="error in (no error)", VISA resource name=w5) -> (VISA resource name=w1:refnum<visa-resource-name>, error out=w2:errorcluster)  [unwired: 2 in]
  n97 = while {
    tunnel: w7 -> [_]
    tunnel: "String" -> [_]
    shift-right: [w296] -> _
    shift-left: w2 -> [w299]
    shift-right: _ -> [_]
    shift-left: "Cluster" -> [w290]
    shift-right: _ -> [_]
    shift-left: w1 -> [w291]
    stop <- w292 stop-if-true
    n98 = VISA Read(VISA resource name=w291, byte count=u32 100, error in (no error)=w299) -> (read buffer=w297:string, error out=w301:errorcluster)  [unwired: 2 out]
    n99 = Wait (ms)(milliseconds to wait=u32 1) -> ()  [unwired: 1 out]
    n100 = xnode "Match Regular Expression"("input string"=w297, "regular expression"="\\[[a-z]+:[0-9A-F]+\\]", "error in"=w301) -> ("whole match"=w293:string, "error out"=w294:errorcluster)  [unwired: 3 in, 3 out]
    n101 = call "LPCA Interface Front Panel Update (Sub-Vi).vi"("error in (no error)"=w294, "regular expression"=w297, "VISA resource name"=w293, "Cluster"=w290) -> ("error out"=w296:errorcluster)  [unwired: 6 in, 1 out]
    n102 = local read "Stop?"() -> (w292:bool)
  }
